vi "split and merge test.vi"() -> ()   [LabVIEW 2017]
panel:
  in  "stop":bool
  out "XY Graph":cluster{dbl[], dbl[]}(graph)
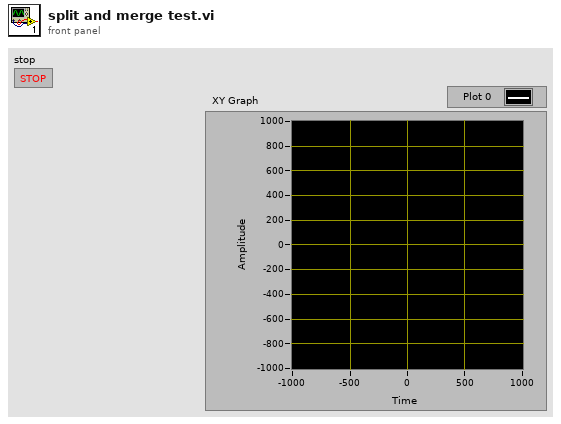
[diagram p1: front panel]
types:
  T1 = typedef "LidarPoint.ctl" = cluster{"X":dbl, "Y":dbl}
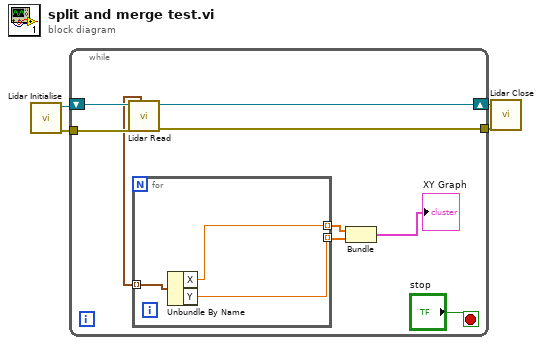
[diagram p0: block diagram]
diagram:
  n1 = call "Lidar Initialise.vi"() -> ("error out"=w2:errorcluster, "VISA resource name out"=w4:refnum<visa-resource-name>)  [unwired: 10 in]
  n2 = while {
    shift-right: [w12] -> w3
    shift-left: w4 -> [w13]
    tunnel: w2 -> [w11]
    tunnel: [w10] -> w1
    stop <- "stop" stop-if-true
    n3 = call "Lidar Read.vi"("error in (no error)"=w11, "VISA resource name"=w13) -> ("error out"=w10:errorcluster, "VISA resource name out"=w12:refnum<visa-resource-name>, "XYflipped"=w8:T1[])  [unwired: 4 in, 2 out]
    n4 = for {
      tunnel: w8 -> [w16] mode=indexing
      tunnel: [w15] -> w6 mode=indexing
      tunnel: [w14] -> w7 mode=indexing
      n5 = Unbundle By Name(w16) -> ("X"=w15:dbl, "Y"=w14:dbl)
    }
    n6 = Bundle(w6, w7) -> (→"XY Graph":cluster{dbl[], dbl[]})  [unwired: 1 in]
  }
  n7 = call "Lidar Close.vi"("error in (no error)"=w1, "VISA resource name"=w3) -> ()  [unwired: 9 in, 1 out]
